vi "restoreDefaultSettings.vi"(8 "error in (no error)":errorcluster, 11 "pHandle":u32) -> (0 "error out":errorcluster, 3 "return type":i32)   [LabVIEW 2011, in "sbgLabView.lvlib"]
uses:
  sbgLabView.lvlib
  sbgMatLab.dll
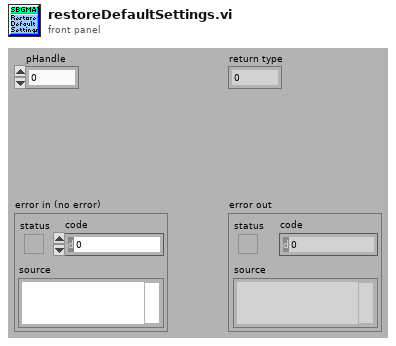
[diagram p1: front panel]
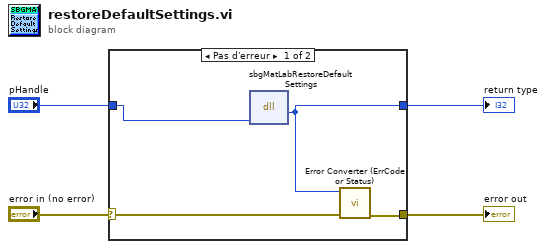
[diagram p0: block diagram]
diagram:
  n1 = case shown="Pas d'erreur" "error in (no error)" {
    selector: "error in (no error)" -> [w6 w9]
    tunnel: [w5 w9] -> w3
    tunnel: [w8 _] -> w2
    tunnel: "pHandle" -> [w7 _]
    frame No Error {
      n2 = dll-call lib="C:/SBG-Systems/remote/projects/software/projects/labviewExample/sbgLabView/sbgMatLab.*" fn="sbgMatLabRestoreDefaultSettings"("pHandle"=w7) -> ("type de retour"=w8:i32)  [unwired: 4 in, 2 out]
      n3 = call "Error Converter (ErrCode or Status).vi"("error in (no error)"=w6, "error code"=w8) -> ("error out"=w5:errorcluster)  [unwired: 9 in]
    }
    frame Error {
    }
  }
  "return type" <- w2
  "error out" <- w3
